vi "9870 Interface Interrupt (FPGA).vi"() -> ()   [LabVIEW 2022 SP3]
uses:
  <vilib>/eio/EIOMethodNode/EIOMethodNode.xnode
  <vilib>/rvi/eio/common/nirviEmuTemplateMethod_errors.vi
  FPGA Function.ctl
panel:
  out "EOS?":bool
  in  "EOS Enabled":bool
  in  "EOS":u8
  in  "Byte Timeout":i32=100
  out "Timed Out Read":bool
  in  "Op Control":T1
  out "Timed Out Write":bool
  out "error out":errorcluster
  out "Byte read":u8 format="%02x"
  in  "Byte to Write":u8 format="%02x"
  # "WRITE"
  # "READ"
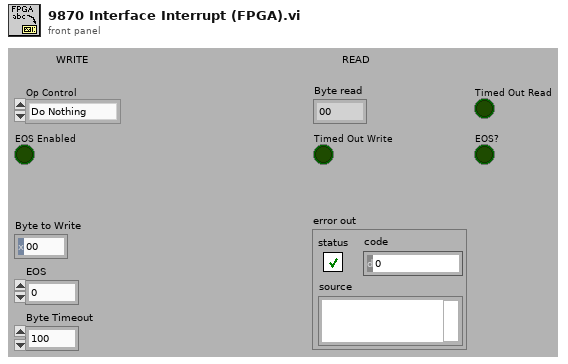
[diagram p1: front panel]
types:
  T1 = typedef "FPGA Function.ctl" = enum16{"Do Nothing", "Write", "Read"}
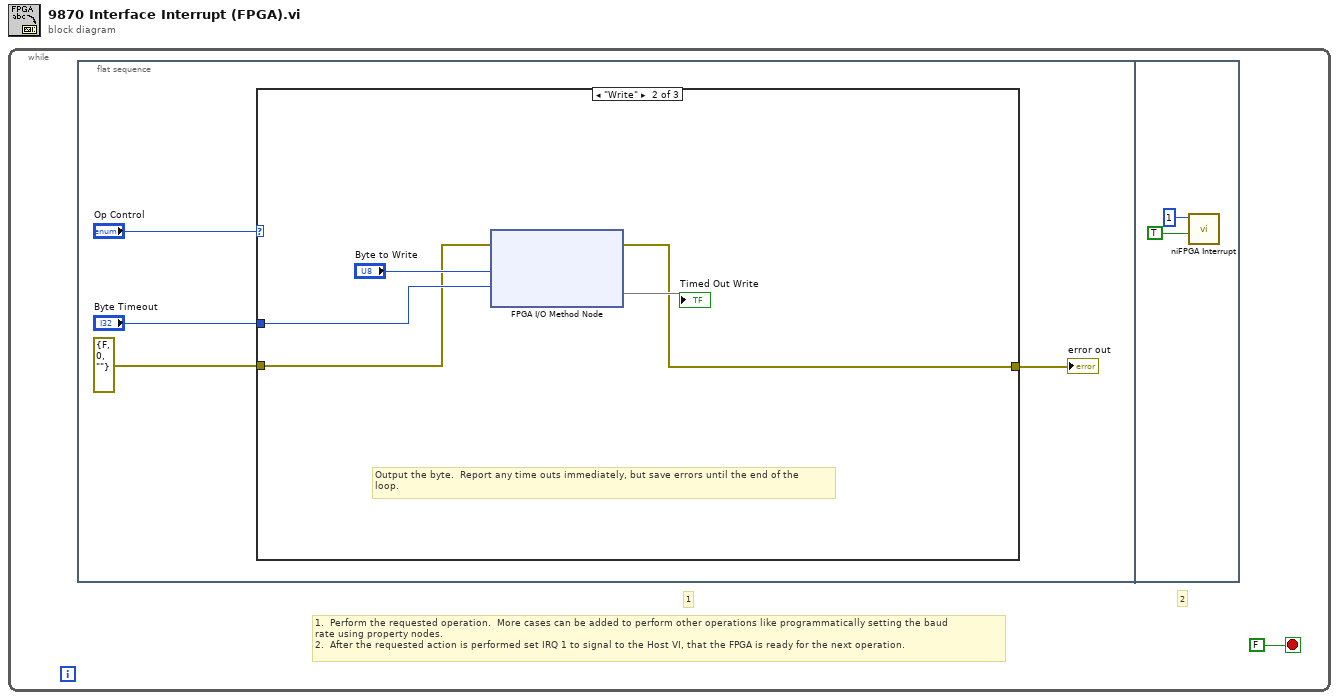
[diagram p0: block diagram]
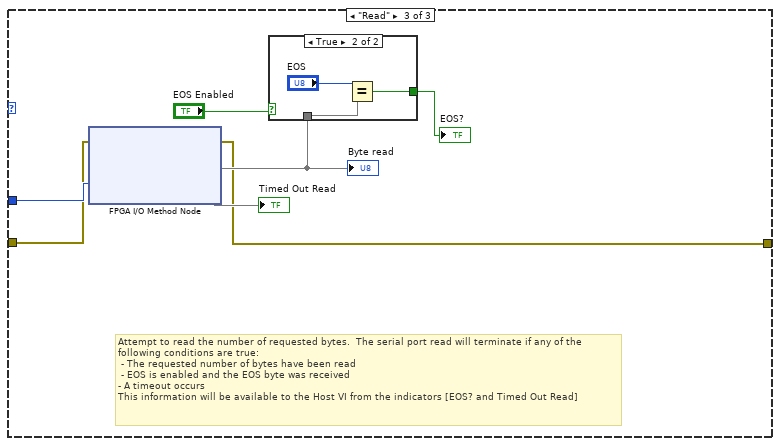
[diagram p3: hidden frame]
diagram:
  n1 = while {
    stop <- FALSE stop-if-true
    # "1.  Perform the requested operation.  More cases can be added to perform other operations like programmatically setting the baud \nrate using property nodes.\n2.  After the requested action is performed set IRQ 1 to signal to the Host VI, that the FPGA is ready for the next operation."
    # "2"
    # "1"
    n2 = flat-sequence {
      frame #0 {
        n3 = case shown="\"Write\"" "Op Control" {
          tunnel: "Byte Timeout" -> [_ w11 w18]
          tunnel: [w6 w7 w12] -> w4
          tunnel: errorcluster {"status"=FALSE, "code"=0, "source"=""} ("error out") -> [w6 w8 w13]
          frame "Do Nothing", Default {
          }
          frame "Write" {
            # "Output the byte.  Report any time outs immediately, but save errors until the end of the\nloop."
            n4 = xnode "FPGA I/O Method Node"("error in"=w8, "Data"="Byte to Write", "Timeout (ms)"=w11) -> ("error out"=w7:errorcluster, "Timed Out"=→"Timed Out Write")  [unwired: 1 in, 1 out]
          }
          frame "Read" {
            # "Attempt to read the number of requested bytes.  The serial port read will terminate if any of the \nfollowing conditions are true:\n - The requested number of bytes have been read\n - EOS is enabled and the EOS byte was received\n- A timeout occurs\nThis information will be available to the Host VI from the indicators [EOS? and Timed Out Read]"
            n5 = xnode "FPGA I/O Method Node"("error in"=w13, "Timeout (ms)"=w18) -> ("error out"=w12:errorcluster, "Data"=w15, "Timed Out"=→"Timed Out Read")  [unwired: 1 in, 1 out]
            "Byte read" <- w15
            n6 = case shown="True" "EOS Enabled" {
              selector: "EOS Enabled" -> [w19 _]
              tunnel: w15 -> [_ w22]
              tunnel: [w19 w20] -> w16
              frame False {
              }
              frame True {
                n7 = Equal?(x="EOS", y=w22) -> (x = y?=w20:bool)
              }
            }
            "EOS?" <- w16
          }
        }
        "error out" <- w4
      }
      frame #1 {
        n8 = call <vilib>:"niFPGA Interrupt.vi"("Wait Until Cleared (F)"=TRUE ("Wait Until Cleared"), "IRQ Number (0)"=u8 1 ("IRQ Number")) -> ()  [unwired: 1 in]
      }
    }
  }
